vi "Delete RPC Client Method Template Files.vi"(8 "error in (no error)":errorcluster, 11 "LVClassLibrary in":refnum<vi>) -> (0 "error out":errorcluster, 3 "LVClassLibrary out":refnum<vi>)   [LabVIEW 2019, in "gRPC Scripting Tools.lvlib"]
uses:
  gRPC Scripting Tools.lvlib
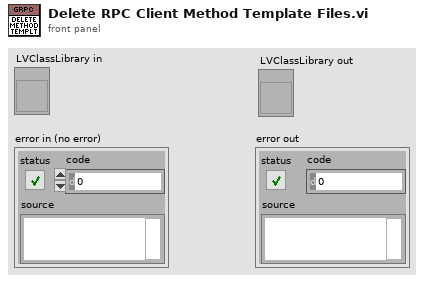
[diagram p1: front panel]
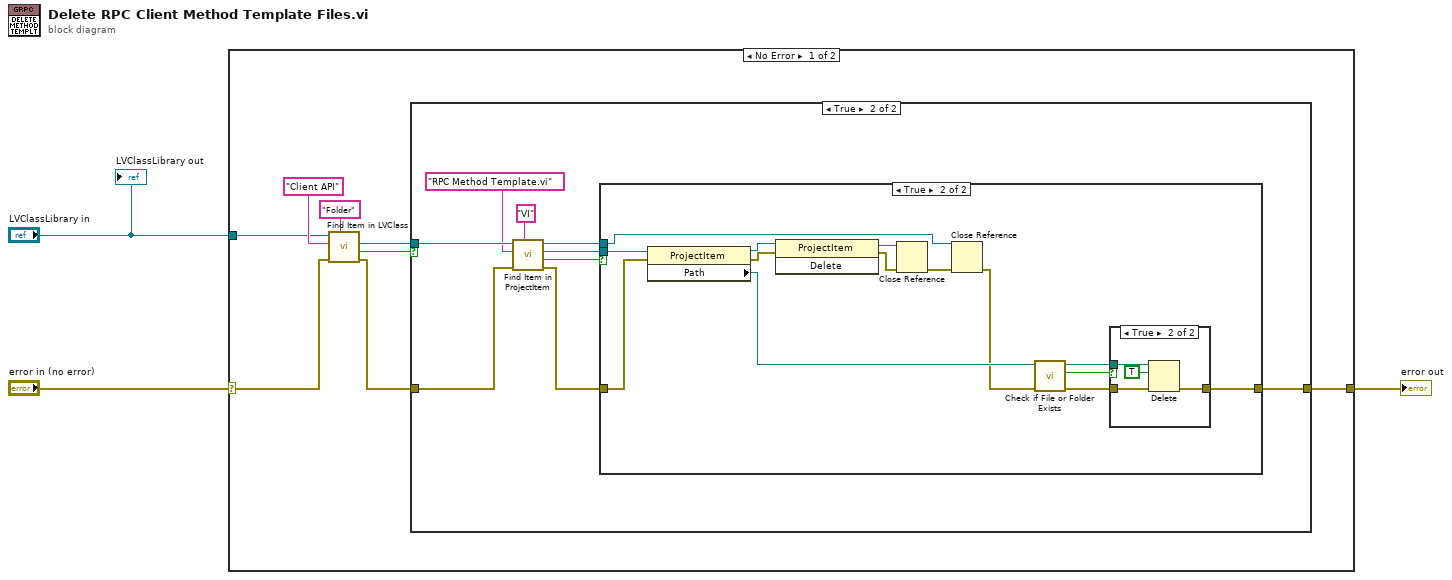
[diagram p0: block diagram]
diagram:
  n1 = case shown="No Error" "error in (no error)" {
    selector: "error in (no error)" -> [w5 w42]
    tunnel: "LVClassLibrary in" -> [w9 _]
    tunnel: [w4 w42] -> w1
    frame No Error {
      n2 = call "Find Item in LVClass.vi"("Item Type"="Folder", "error in (no error)"=w5, "Item Name"="Client API", "Class Item in"=w9) -> ("error out"=w7:errorcluster, "Found?"=w6:bool, "Project Item (Class Item)"=w8:refnum<vi>)  [unwired: 4 in, 1 out]
      n3 = case shown="True" w6 {
        tunnel: w8 -> [_ w21]
        tunnel: w7 -> [w12 w15]
        tunnel: [w12 w13] -> w4
        frame False {
        }
        frame True {
          n4 = call "Find Item in ProjectItem.vi"("Item Type"="VI", "error in (no error)"=w15, "Name"="RPC Method Template.vi" ("Item Type"), "ProjectItem in"=w21) -> ("error out"=w14:errorcluster, "Found ?"=w18:bool, "Item Refnum out"=w16:refnum<vi>, "ProjectItem out"=w17:refnum<vi>)  [unwired: 4 in]
          n5 = case shown="True" w18 {
            tunnel: w14 -> [w22 w36]
            tunnel: w16 -> [_ w35]
            tunnel: w17 -> [_ w24]
            tunnel: [w22 w30] -> w13
            frame False {
            }
            frame True {
              n6 = property class="ProjectItem"(reference=w35, error in=w36) -> (reference out=w27:refnum<vi>, error out=w28:errorcluster, "Path"=w31:path)
              n7 = invoke class="ProjectItem" method="Delete"(reference=w27, error in=w28) -> (reference out=w29:refnum<vi>, error out=w23:errorcluster)  [unwired: 1 in, 1 out]
              n8 = Close Reference(reference=w29, error in (no error)=w23) -> (error out=w26:errorcluster)
              n9 = Close Reference(reference=w24, error in (no error)=w26) -> (error out=w25:errorcluster)
              n10 = call <vilib>:"Check if File or Folder Exists.vi"("error in (no error)"=w25, "path"=w31) -> ("error out"=w34:errorcluster, "file or folder exists?"=w32:bool, "dup path"=w33:path)  [unwired: 7 in]
              n11 = case shown="True" w32 {
                tunnel: w33 -> [_ w41]
                tunnel: w34 -> [w37 w40]
                tunnel: [w37 w39] -> w30
                frame False {
                }
                frame True {
                  n12 = Delete(path (use dialog)=w41, entire hierarchy (F)=TRUE, error in=w40) -> (error out=w39:errorcluster)  [unwired: 2 in, 2 out]
                }
              }
            }
          }
        }
      }
    }
    frame Error {
    }
  }
  "error out" <- w1
  "LVClassLibrary out" <- "LVClassLibrary in"
